vi "CapturaImagenyQR_subVI_pruebas.vi"(8 "error in (no error)":errorcluster) -> (0 "error out":errorcluster, 2 "código leído?":bool, 3 "Datos_QR":string)   [LabVIEW 2019]
uses:
  <vilib>/vision/Instrument.llb/QR Code Search Options.ctl
  <vilib>/vision/Instrument.llb/Demodulation Mode.ctl
  <vilib>/vision/Instrument.llb/Cell Sample Size.ctl
  <vilib>/vision/Instrument.llb/Cell Filter Mode.ctl
  <vilib>/vision/Instrument.llb/QR Code Description Options.ctl
  <vilib>/vision/Instrument.llb/Data Matrix Polarity.ctl
  <vilib>/vision/Instrument.llb/QR Code Model Type.ctl
  <vilib>/vision/NI_Vision_Development_Module.lvlib
panel:
  out "path":path=path "C:/Trabajo_Robot/desde Marzo 2023/Pruebas_PC_APD/Ficher_LabView/capturaQR.jpg"
  in  "DNVideoX":refnum<k7>(container)
  # "Esta VI borra el fichero previo con la imagen de la superficie del código QR,\ny genera otra imagen nueva para el ASIC colocado en el socket, pero NO hace una \ncomprobación del borde o marco alrrededor del código QR del ASIC."
  # "Captura una imagen que guarda como \"CapturaQR.jpg\" en el directorio antes mencionado \n arriba y después accede a esa imagen para leer el código QR (y lo devuelve como un string)."
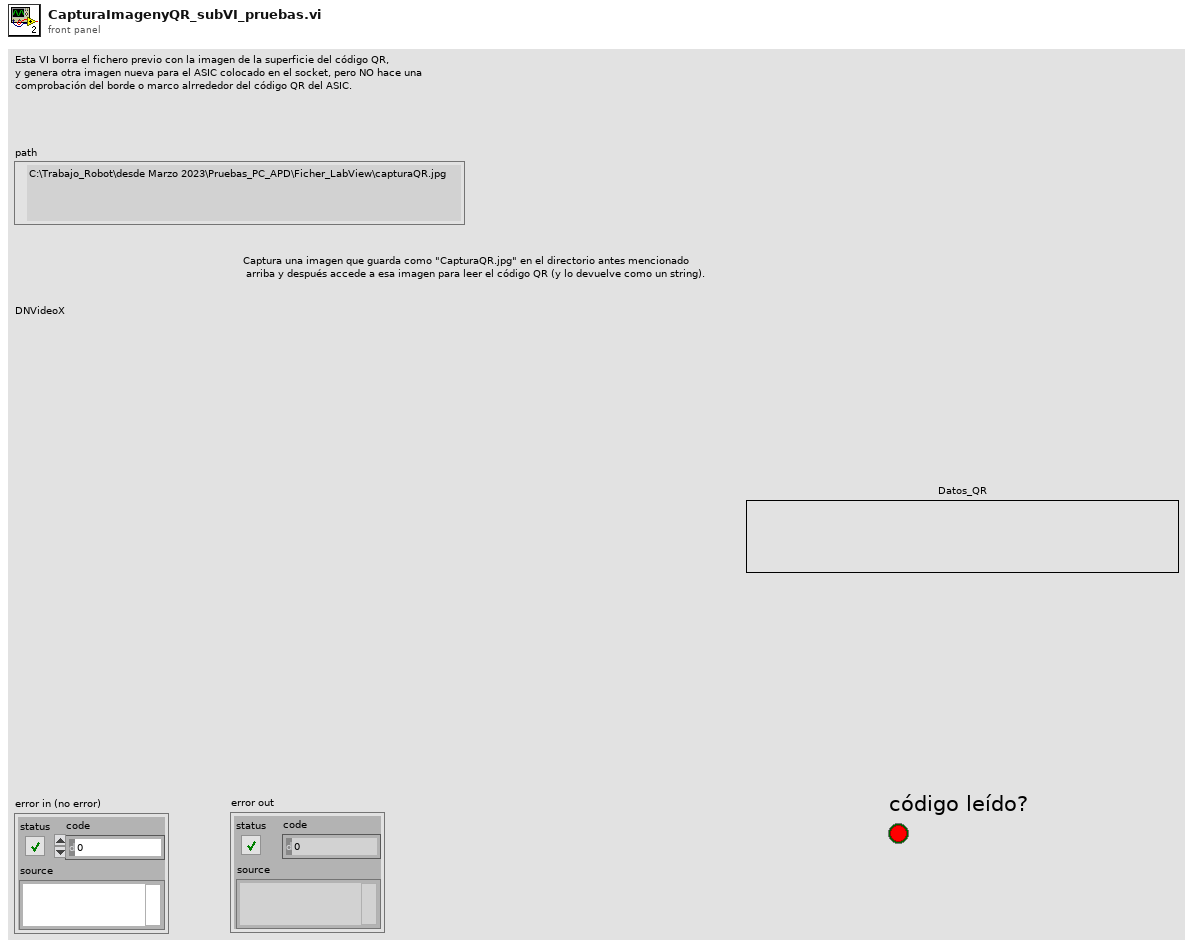
[diagram p1: front panel]
types:
  T1 = typedef "QR Code Description Options.ctl" = cluster{"Matrix Size (cells)":i32, "Barcode Polarity":T2, "Mirror Mode":i32, "QR Model":T3}
  T2 = typedef "Data Matrix Polarity.ctl" = i32
  T3 = typedef "QR Code Model Type.ctl" = i32
  T4 = typedef "QR Code Search Options.ctl" = cluster{"Rotation Mode":enum32{"Unlimited", "0 Degrees", "90 Degrees", "180 Degrees", "270 Degrees"}, "Skip Location?":bool, "Edge Threshold":u32, "Demodulation Mode":T5, "Cell Sample Size":T6, "Cell Filter Mode":T7, "Skew Degrees Allowed":u32}
  T5 = typedef "Demodulation Mode.ctl" = i32
  T6 = typedef "Cell Sample Size.ctl" = i32
  T7 = typedef "Cell Filter Mode.ctl" = i32
  T8 = cluster{"Brightness":sgl, "Contrast":sgl, "Gamma":sgl}
  T9 = typedef "IMAQ Image.ctl" = refnum<image>
  T10 = typedef "QR Code Report.ctl" = cluster{"Found?":bool, "Data":string, "Bounding Box":cluster{"x":sgl, "y":sgl}[], "Errors Corrected":u32, "Dimensions (Rows/Cols)":u32, "Version":u32, "QR Model":T3, "Stream Mode":T11, "Barcode Polarity":T2, "Mirrored?":bool, "Append Stream Position":u32, "Size of Append Stream":u32, "First EAN-128 ID":i32, "First Alternate Language ID":i32, "Append Stream ID":u32, "Minimum Edge Strength":u32, "Demodulation Mode":T5, "Cell Sample Size":T6, "Cell Filter Mode":T7}
  T11 = typedef "QR Code Stream Mode Type.ctl" = i32
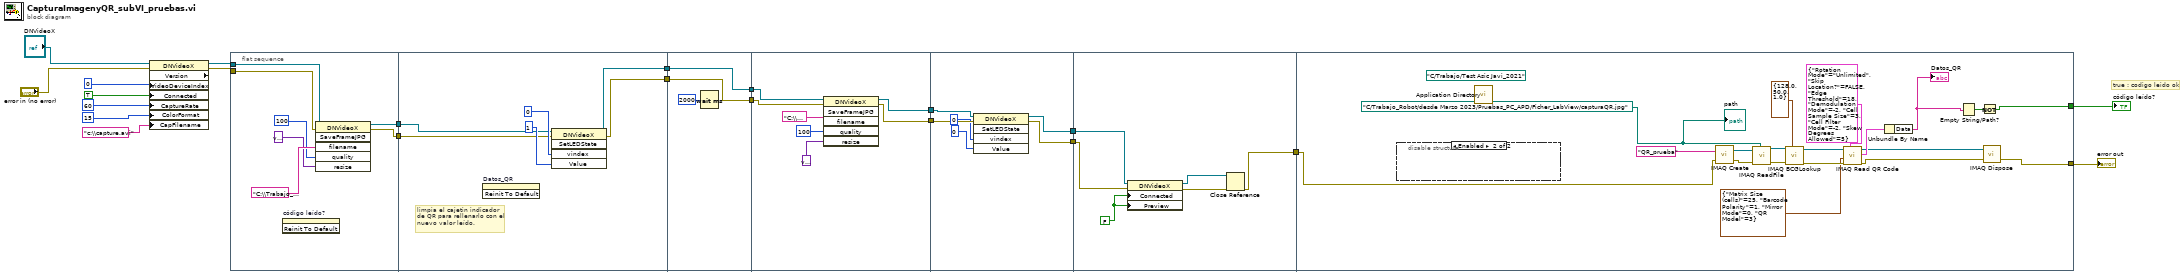
[diagram p0: block diagram]
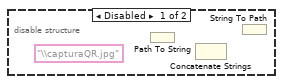
[diagram p2: hidden frame]
diagram:
  # "true : codigo leido ok"
  n1 = property class="DNVideoX" props=["Version", "VideoDeviceIndex", "Connected", "CaptureRate", "ColorFormat", "CapFilename"](reference="DNVideoX", error in="error in (no error)", "VideoDeviceIndex"=0, "Connected"=TRUE, "CaptureRate"=60 ("VideoDeviceIndex"), "ColorFormat"=15 ("VideoDeviceIndex"), "CapFilename"="c:\\capture.avi" ("default name")) -> (reference out=w3:refnum<k7>, error out=w2:errorcluster)  [unwired: 1 out]
  n2 = flat-sequence {
    tunnel: w3 -> [w26]
    tunnel: w2 -> [w25]
    tunnel: [w23] -> w19
    tunnel: [w24] -> w18
    tunnel: w19 -> [w31]
    tunnel: [w35] -> w17
    tunnel: [w34] -> w16
    tunnel: w18 -> [w30]
    tunnel: w17 -> [w37]
    tunnel: w16 -> [w36]
    tunnel: [w37] -> w15
    tunnel: [w36] -> w14
    tunnel: w15 -> [w43]
    tunnel: w14 -> [w39]
    tunnel: [w41] -> w13
    tunnel: [w40] -> w12
    tunnel: w13 -> [w47]
    tunnel: w12 -> [w51]
    tunnel: [w46] -> w11
    tunnel: [w50] -> w10
    tunnel: w11 -> [w53]
    tunnel: w10 -> [w55]
    tunnel: [w52] -> w9
    tunnel: w9 -> [w62]
    tunnel: [w61] -> w21
    tunnel: [w58] -> w1
    frame #0 {
      n3 = invoke on="código leído?" class="Bool (strict)" method="Reinit To Default"() -> ()  [unwired: 3 in, 3 out]
      n4 = invoke class="DNVideoX" method="SaveFrameJPG"(reference=w26, error in=w25, "filename"="C:\\Trabajo_Robot\\desde Marzo 2023\\Pruebas_PC_APD\\Ficher_LabView\\capturaQR.jpg", "quality"=100, "resize"=variant) -> (reference out=w24:refnum<k7>, error out=w23:errorcluster)  [unwired: 1 in, 4 out]
    }
    frame #1 {
      # "limpia el cajetin indicador\nde QR para rellenarlo con el \nnuevo valor leído."
      n5 = invoke on="Datos_QR" class="Str" method="Reinit To Default"() -> ()  [unwired: 3 in, 3 out]
      n6 = invoke class="DNVideoX" method="SetLEDState"(reference=w30, error in=w31, "vindex"=0, "Value"=1) -> (reference out=w35:refnum<k7>, error out=w34:errorcluster)  [unwired: 1 in, 3 out]
    }
    frame #2 {
      n7 = Wait (ms)(milliseconds to wait=u32 2000) -> ()  [unwired: 1 out]
    }
    frame #3 {
      n8 = invoke class="DNVideoX" method="SaveFrameJPG"(reference=w43, error in=w39, "filename"="C:\\Trabajo_Robot\\desde Marzo 2023\\Pruebas_PC_APD\\Ficher_LabView\\capturaQR.jpg", "quality"=100, "resize"=variant) -> (reference out=w41:refnum<k7>, error out=w40:errorcluster)  [unwired: 1 in, 4 out]
    }
    frame #4 {
      n9 = invoke class="DNVideoX" method="SetLEDState"(reference=w47, error in=w51, "vindex"=0, "Value"=0) -> (reference out=w46:refnum<k7>, error out=w50:errorcluster)  [unwired: 1 in, 3 out]
    }
    frame #5 {
      w54 = FALSE ("Connected")
      n10 = property class="DNVideoX"(reference=w53, error in=w55, "Connected"=w54, "Preview"=w54) -> (reference out=w56:refnum<k7>, error out=w57:errorcluster)
      n11 = Close Reference(reference=w56, error in (no error)=w57) -> (error out=w52:errorcluster)
    }
    frame #6 {
      w65 = path "C:/Trabajo_Robot/desde Marzo 2023/Pruebas_PC_APD/Ficher_LabView/capturaQR.jpg" ("path")
      (unwired) path "C:/Trabajo/Test Asic Javi_2021" ("path 2")
      n12 = disable-structure shown="Enabled" {
        frame Disabled {
          (unwired) "\\capturaQR.jpg" ("Image Name")
          n13 = Path To String() -> ()  [unwired: 1 in, 1 out]
          n14 = Concatenate Strings() -> ()  [unwired: 2 in, 1 out]
          n15 = String To Path() -> ()  [unwired: 1 in, 1 out]
        }
        frame Enabled {
        }
      }
      n16 = call <vilib>:"Application Directory.vi"() -> ()  [unwired: 1 out]
      n17 = call "IMAQ Create"("Image Name"="QR_prueba", "error in (no error)"=w62) -> ("New Image"=w66:T9, "error out"=w67:errorcluster)  [unwired: 3 in]
      n18 = call "IMAQ ReadFile"("File Path"=w65, "error in (no error)"=w67, "Image"=w66) -> ("error out"=w74:errorcluster, "Image Out"=w70:T9)  [unwired: 4 in, 3 out]
      n19 = call "IMAQ BCGLookup"("Image Src"=w70, "BCG Values"=T8 {"Brightness"=128.0, "Contrast"=50.0, "Gamma"=1.0}, "error in (no error)"=w74) -> ("Image Dst Out"=w75:T9, "error out"=w76:errorcluster)  [unwired: 4 in]
      n20 = call "IMAQ Read QR Code"("QR Search Options"=T4 {"Rotation Mode"=enum."Unlimited", "Skip Location?"=FALSE, "Edge Threshold"=18, "Demodulation Mode"=-2, "Cell Sample Size"=3, "Cell Filter Mode"=-2, "Skew Degrees Allowed"=5}, "error in (no error)"=w76, "QR Description Options"=T1 {"Matrix Size (cells)"=25, "Barcode Polarity"=1, "Mirror Mode"=0, "QR Model"=3}, "Image"=w75) -> ("error out"=w64:errorcluster, "QR Code Report"=w73:T10, "Image (duplicate)"=w63:T9)  [unwired: 4 in, 1 out]
      n21 = Unbundle By Name(w73) -> ("Data"=w60:string)
      "Datos_QR" <- w60
      n22 = Empty String/Path?(string/path=w60) -> (empty?=w59:bool)
      n23 = Not(x=w59) -> (.not. x?=w58:bool)
      n24 = call "IMAQ Dispose"("Image"=w63, "error in (no error)"=w64) -> ("error out"=w61:errorcluster)  [unwired: 4 in]
      "path" <- w65
    }
  }
  "error out" <- w21
  "código leído?" <- w1
